vi "destroyEvents.vi"(8 "error in (no error)":errorcluster, 11 "CameraEventsManger in":refnum<class "CameraEventsManger.lvclass">) -> (0 "error out":errorcluster, 3 "CameraEventsManger out":refnum<class "CameraEventsManger.lvclass">)   [LabVIEW 2011, in "Tools.lvlib" / "Settings.lvlib" / "CameraEventsManger.lvclass"]
uses:
  CameraEventsManger.lvclass
  CameraEventsManger.lvclass/CameraEventsManger.ctl
  Viewers/Snapper/SnapperEvents.lvclass
  Tools/SettingsEventManager/SettingsEventsManager.lvclass
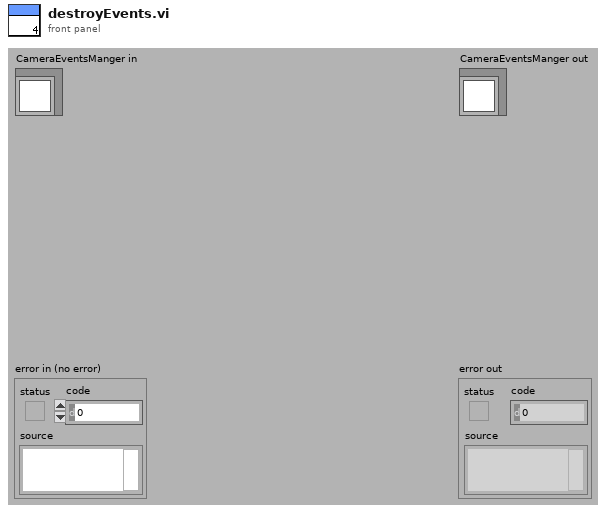
[diagram p1: front panel]
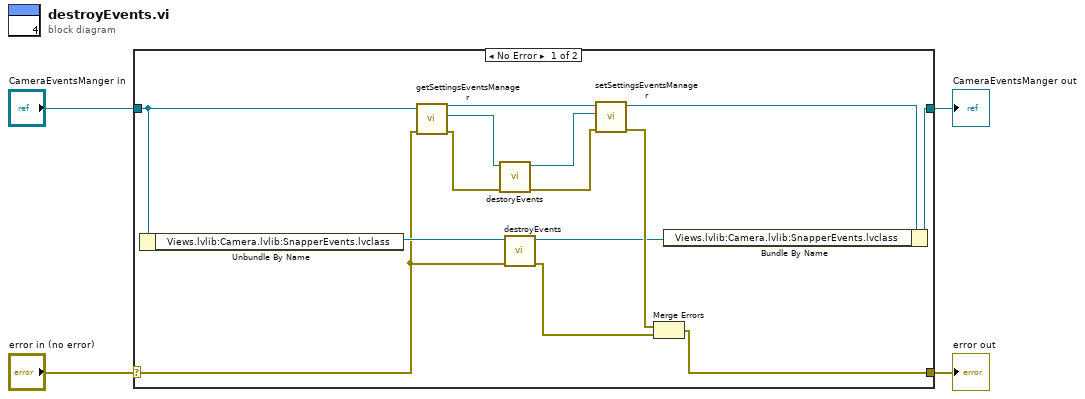
[diagram p0: block diagram]
diagram:
  n1 = case shown="No Error" "error in (no error)" {
    selector: "error in (no error)" -> [w11 w20]
    tunnel: [w8 w20] -> w3
    tunnel: [w6 w19] -> w1
    tunnel: "CameraEventsManger in" -> [w13 w19]
    frame No Error {
      n2 = Unbundle By Name(w13) -> ("Views.lvlib:Camera.lvlib:SnapperEvents.lvclass"=w12:refnum<class "SnapperEvents.lvclass">)
      n3 = call-dynamic "getSettingsEventsManager.vi"("error in (no error)"=w11, "CameraEventsManger.lvclass in"=w13) -> ("error out"=w17:errorcluster, "SettingsEventsManager"=w18:refnum<class "SettingsEventsManager.lvclass">, "CameraEventsManger.lvclass out"=w16:refnum<class "CameraEventsManger.lvclass">)  [unwired: 7 in]
      n4 = call-dynamic "destoryEvents.vi"("error in (no error)"=w17, "SettingsEventsManager in"=w18) -> ("error out"=w14:errorcluster, "SettingsEventsManager out"=w15:refnum<class "SettingsEventsManager.lvclass">)  [unwired: 8 in]
      n5 = call-dynamic "destroyEvents.vi"("error in (no error)"=w11, "SnapperEvents in"=w12) -> ("error out"=w9:errorcluster, "SnapperEvents out"=w5:refnum<class "SnapperEvents.lvclass">)  [unwired: 8 in]
      n6 = call-dynamic "setSettingsEventsManager.vi"("error in (no error)"=w14, "Tools.lvlib:Settings.lvlib:SettingsEventsManager.lvclass"=w15, "CameraEventsManger.lvclass in"=w16) -> ("error out"=w10:errorcluster, "CameraEventsManger.lvclass out"=w7:refnum<class "CameraEventsManger.lvclass">)  [unwired: 7 in]
      n7 = Merge Errors(w10, w9) -> (w8:errorcluster)
      n8 = Bundle By Name(cluster=w7, "Views.lvlib:Camera.lvlib:SnapperEvents.lvclass"=w5) -> (w6:refnum<class "CameraEventsManger.lvclass">)
    }
    frame Error {
    }
  }
  "error out" <- w3
  "CameraEventsManger out" <- w1
